vi "Connection.Properties.vi"(7 "Action":enum8{"Get", "Set"}(ring), 8 "error in (no error)":errorcluster, 10 "Connection.Properties":T1={"Server IP Address"="localhost", "Server Port"=49350, "Message Mode"=enum."None", "Security"=enum."Basic256", "User Name"="", "Password"="", "Client Certificate"=path "", "Server Certificate"=path ""}, 11 "Item Ref in":T2 format="%.0x") -> (0 "error out":errorcluster, 2 "Connection.Properties":T1={"Server IP Address"="localhost", "Server Port"=49350, "Message Mode"=enum."None", "Security"=enum."Basic256", "User Name"="", "Password"="", "Client Certificate"=path "", "Server Certificate"=path ""}, 3 "Item Ref out":T2 format="%.0x")   [LabVIEW 2013, in "OPC UA Client System Explorer.lvlib"]
uses:
  OPC UA Client System Explorer.lvlib
  <vilib>/NI Veristand/Custom Device API/Custom Device Item Ref.ctl
  Shared/Connection.Properties.ctl
  <vilib>/NI Veristand/Custom Device API/Dependent File Optional Info.ctl
  Shared/Constants.vi
  <vilib>/NI Veristand/Custom Device API/Get Item Property (String).vi
  <vilib>/NI Veristand/Custom Device API/Get Item Property (U16).vi
  <vilib>/NI Veristand/Custom Device API/Get Item Property (Dependent File).vi
  <vilib>/NI Veristand/Custom Device API/Set Item Property (String).vi
  <vilib>/NI Veristand/Custom Device API/Set Item Property (U16).vi
  <vilib>/NI Veristand/Custom Device API/Set Item Property (Dependent File).vi
  <vilib>/NI Veristand/Custom Device API/Custom Device API.lvlib
  Shared/OPC UA Client Shared.lvlib
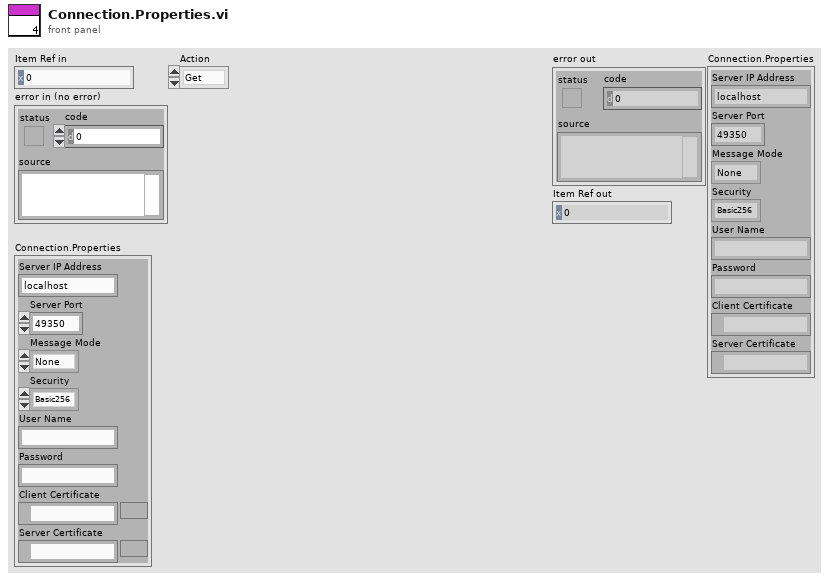
[diagram p1: front panel]
types:
  T1 = typedef "OPC UA Client Shared.lvlib/Connection.Properties.ctl" = cluster{"Server IP Address":string, "Server Port":u16, "Message Mode":enum16{"None", "Sign", "Sign and Encrypt"}, "Security":enum16{"Basic256", "Basic128Rsa15"}, "User Name":string, "Password":string, "Client Certificate":path, "Server Certificate":path}
  T2 = typedef "Custom Device API.lvlib/Custom Device Item Ref.ctl" = u64
  T3 = typedef "Custom Device API.lvlib/Dependent File Optional Info.ctl" = cluster{"Version":string, "RTDestination":path, "ForceDownload":bool, "SupportedTarget":string, "MD5":string}
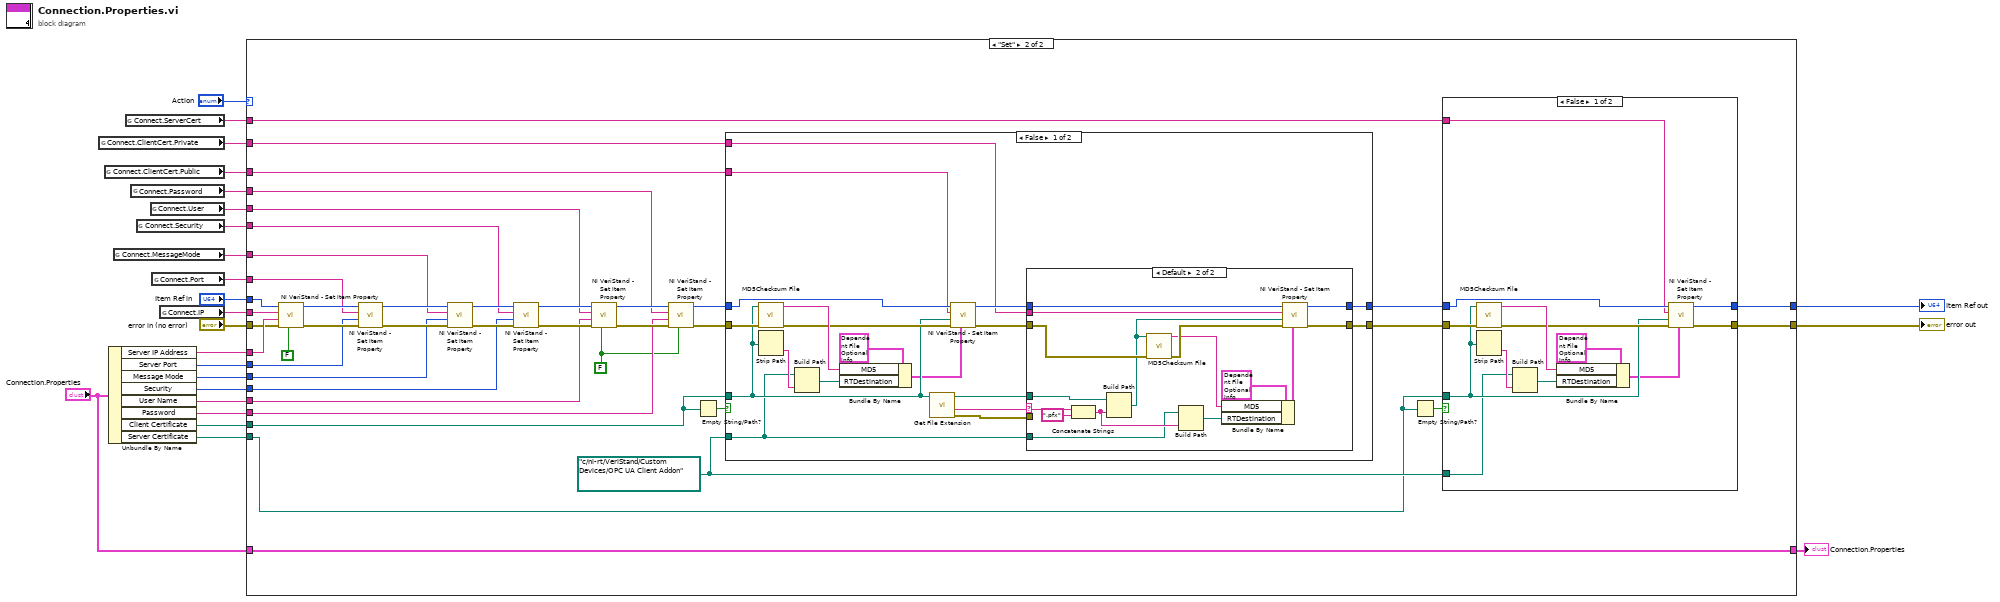
[diagram p0: block diagram]
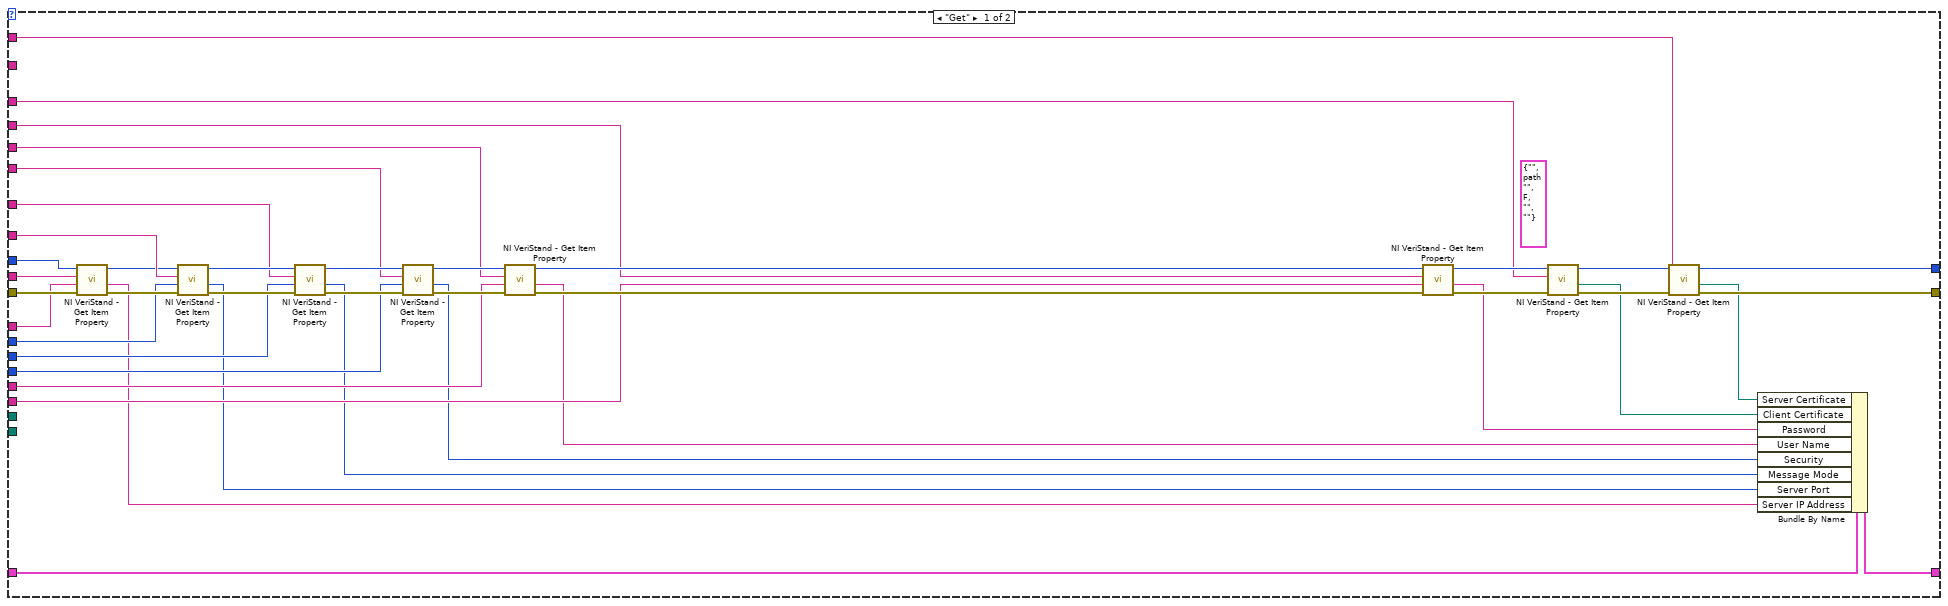
[diagram p2: hidden frame]
diagram:
  n1 = global read "Constants.vi" "Connect.ClientCert.Private"() -> (w15:string)
  n2 = global read "Constants.vi" "Connect.ClientCert.Public"() -> (w14:string)
  n3 = Unbundle By Name("Connection.Properties") -> ("Server IP Address"=w23:string, "Server Port"=w22:u16, "Message Mode"=w21:enum16{"None", "Sign", "Sign and Encrypt"}, "Security"=w20:enum16{"Basic256", "Basic128Rsa15"}, "User Name"=w19:string, "Password"=w18:string, "Client Certificate"=w4:path, "Server Certificate"=w17:path)
  n4 = global read "Constants.vi" "Connect.MessageMode"() -> (w12:string)
  n5 = global read "Constants.vi" "Connect.ServerCert"() -> (w16:string)
  n6 = global read "Constants.vi" "Connect.Password"() -> (w10:string)
  n7 = global read "Constants.vi" "Connect.Security"() -> (w13:string)
  n8 = global read "Constants.vi" "Connect.User"() -> (w11:string)
  n9 = global read "Constants.vi" "Connect.Port"() -> (w5:string)
  n10 = global read "Constants.vi" "Connect.IP"() -> (w24:string)
  n11 = case shown="\"Set\"" "Action" {
    tunnel: w24 -> [w57 w107]
    tunnel: w23 -> [w48 w94]
    tunnel: w22 -> [w47 w93]
    tunnel: w21 -> [w46 w92]
    tunnel: w20 -> [w45 w91]
    tunnel: w19 -> [w44 w90]
    tunnel: w18 -> [w43 w89]
    tunnel: w17 -> [_ w67]
    tunnel: w16 -> [w35 w72]
    tunnel: w15 -> [_ w88]
    tunnel: w14 -> [w36 w87]
    tunnel: w13 -> [w39 w86]
    tunnel: w12 -> [w40 w85]
    tunnel: w11 -> [w38 w84]
    tunnel: w10 -> [w37 w83]
    tunnel: [w42 w70] -> w9
    tunnel: [w41 w71] -> w8
    tunnel: "Item Ref in" -> [w58 w80]
    tunnel: "error in (no error)" -> [w66 w79]
    tunnel: w5 -> [w56 w78]
    tunnel: w4 -> [_ w76]
    tunnel: "Connection.Properties" -> [w34 w77]
    tunnel: [w25 w77] -> w2
    frame "Get" {
      (unwired) T3 {"Version"="", "RTDestination"=path "", "ForceDownload"=FALSE, "SupportedTarget"="", "MD5"=""} ("OptionalInfo")
      n12 = call-poly <vilib>:"NI VeriStand - Get Item Property.vi"("error in (no error)"=w66, "Default Value"=w48, "Property Name"=w57, "Item Ref in"=w58) -> ("error out"=w65:errorcluster, "Value"=w29:string, "Item Ref out"=w55:T2)  [unwired: 4 in, 1 out]
      n13 = call-poly <vilib>:"NI VeriStand - Get Item Property.vi"("error in (no error)"=w65, "Default Value"=w47, "Property Name"=w56, "Item Ref in"=w55) -> ("error out"=w64:errorcluster, "Value"=w28:u16, "Item Ref out"=w54:T2)  [unwired: 4 in, 1 out]
      n14 = call-poly <vilib>:"NI VeriStand - Get Item Property.vi"("error in (no error)"=w64, "Default Value"=w46, "Property Name"=w40, "Item Ref in"=w54) -> ("error out"=w63:errorcluster, "Value"=w27:u16, "Item Ref out"=w53:T2)  [unwired: 4 in, 1 out]
      n15 = call-poly <vilib>:"NI VeriStand - Get Item Property.vi"("error in (no error)"=w63, "Default Value"=w45, "Property Name"=w39, "Item Ref in"=w53) -> ("error out"=w62:errorcluster, "Value"=w26:u16, "Item Ref out"=w52:T2)  [unwired: 4 in, 1 out]
      n16 = call-poly <vilib>:"NI VeriStand - Get Item Property.vi"("error in (no error)"=w62, "Default Value"=w44, "Property Name"=w38, "Item Ref in"=w52) -> ("error out"=w61:errorcluster, "Value"=w30:string, "Item Ref out"=w51:T2)  [unwired: 4 in, 1 out]
      n17 = call-poly <vilib>:"NI VeriStand - Get Item Property.vi"("error in (no error)"=w61, "Default Value"=w43, "Property Name"=w37, "Item Ref in"=w51) -> ("error out"=w60:errorcluster, "Value"=w31:string, "Item Ref out"=w50:T2)  [unwired: 4 in, 1 out]
      n18 = call-poly <vilib>:"NI VeriStand - Get Item Property.vi"("error in (no error)"=w60, "Property Name"=w36, "Item Ref in"=w50) -> ("error out"=w59:errorcluster, "Path"=w32:path, "Item Ref out"=w49:T2)  [unwired: 4 in, 2 out]
      n19 = call-poly <vilib>:"NI VeriStand - Get Item Property.vi"("error in (no error)"=w59, "Property Name"=w35, "Item Ref in"=w49) -> ("error out"=w42:errorcluster, "Path"=w33:path, "Item Ref out"=w41:T2)  [unwired: 4 in, 2 out]
      n20 = Bundle By Name(cluster=w34, "Server Certificate"=w33, "Client Certificate"=w32, "Password"=w31, "User Name"=w30, "Security"=w26, "Message Mode"=w27, "Server Port"=w28, "Server IP Address"=w29) -> (w25:T1)
    }
    frame "Set" {
      w69 = path "c:/ni-rt/VeriStand/Custom Devices/OPC UA Client Addon" ("RTDestination")
      w82 = FALSE ("Binary String (T)")
      n21 = call-poly <vilib>:"NI VeriStand - Set Item Property.vi"("Binary String (T)"=FALSE, "error in (no error)"=w79, "Value"=w94, "Property Name"=w107, "Item Ref in"=w80) -> ("error out"=w100:errorcluster, "Item Ref out"=w106:T2)  [unwired: 4 in, 1 out]
      n22 = call-poly <vilib>:"NI VeriStand - Set Item Property.vi"("error in (no error)"=w100, "Value"=w93, "Property Name"=w78, "Item Ref in"=w106) -> ("error out"=w99:errorcluster, "Item Ref out"=w105:T2)  [unwired: 5 in, 1 out]
      n23 = call-poly <vilib>:"NI VeriStand - Set Item Property.vi"("error in (no error)"=w99, "Value"=w92, "Property Name"=w85, "Item Ref in"=w105) -> ("error out"=w98:errorcluster, "Item Ref out"=w104:T2)  [unwired: 5 in, 1 out]
      n24 = call-poly <vilib>:"NI VeriStand - Set Item Property.vi"("error in (no error)"=w98, "Value"=w91, "Property Name"=w86, "Item Ref in"=w104) -> ("error out"=w97:errorcluster, "Item Ref out"=w103:T2)  [unwired: 5 in, 1 out]
      n25 = call-poly <vilib>:"NI VeriStand - Set Item Property.vi"("Binary String (T)"=w82, "error in (no error)"=w97, "Value"=w90, "Property Name"=w84, "Item Ref in"=w103) -> ("error out"=w96:errorcluster, "Item Ref out"=w102:T2)  [unwired: 4 in, 1 out]
      n26 = call-poly <vilib>:"NI VeriStand - Set Item Property.vi"("Binary String (T)"=w82, "error in (no error)"=w96, "Value"=w89, "Property Name"=w83, "Item Ref in"=w102) -> ("error out"=w95:errorcluster, "Item Ref out"=w101:T2)  [unwired: 4 in, 1 out]
      n27 = Empty String/Path?(string/path=w76) -> (empty?=w75:bool)
      n28 = case shown="False" w75 {
        tunnel: w101 -> [w141 w160]
        tunnel: w95 -> [w127 w161]
        tunnel: [w139 w160] -> w73
        tunnel: w88 -> [w138 _]
        tunnel: w87 -> [w137 _]
        tunnel: [w135 w161] -> w74
        tunnel: w76 -> [w125 _]
        tunnel: w69 -> [w123 _]
        frame False {
          n29 = call <vilib>:"MD5Checksum File.vi"("error in (no error)"=w127, "Path"=w125) -> ("error out"=w126:errorcluster, "MD5 message-digest"=w128:string)  [unwired: 8 in]
          n30 = Strip Path(path=w125) -> (name=w130:string)  [unwired: 1 out]
          n31 = Build Path(base path=w123, name or relative path=w130) -> (appended path=w131:path)
          n32 = Bundle By Name(cluster=T3 {"Version"="1.0", "RTDestination"=path "c:/ni-rt/VeriStand/Custom Devices/FPGA Addon", "ForceDownload"=FALSE, "SupportedTarget"="All", "MD5"=""} ("OptionalInfo"), "MD5"=w128, "RTDestination"=w131) -> (w124:T3)
          n33 = call <vilib>:"Get File Extension.vi"("file"=w125) -> ("error out"=w133:errorcluster, "filename without extension"=w134:string, "dup file"=w132:path)  [unwired: 7 in, 1 out]
          n34 = call-poly <vilib>:"NI VeriStand - Set Item Property.vi"("OptionalInfo"=w124, "error in (no error)"=w126, "Path"=w125, "Property Name"=w137, "Item Ref in"=w141) -> ("error out"=w136:errorcluster, "Item Ref out"=w140:T2)  [unwired: 4 in, 1 out]
          n35 = case shown="Default" w134 {
            selector: w134 -> [_ w155]
            tunnel: w140 -> [w142 w159]
            tunnel: [w142 w158] -> w139
            tunnel: w138 -> [_ w157]
            tunnel: w136 -> [w143 w152]
            tunnel: [w143 w156] -> w135
            tunnel: w133 -> [_ _]
            tunnel: w132 -> [_ w153]
            tunnel: w123 -> [_ w144]
            frame "" {
            }
            frame Default {
              n36 = Concatenate Strings(w155, ".pfx" ("string")) -> (w145:string)
              n37 = Build Path(base path=w153, name or relative path=w145) -> (appended path=w146:path)
              n38 = call <vilib>:"MD5Checksum File.vi"("error in (no error)"=w152, "Path"=w146) -> ("error out"=w151:errorcluster, "MD5 message-digest"=w148:string)  [unwired: 8 in]
              n39 = Build Path(base path=w144, name or relative path=w145) -> (appended path=w149:path)
              n40 = Bundle By Name(cluster=T3 {"Version"="1.0", "RTDestination"=path "c:/ni-rt/VeriStand/Custom Devices/FPGA Addon", "ForceDownload"=FALSE, "SupportedTarget"="All", "MD5"=""} ("OptionalInfo"), "MD5"=w148, "RTDestination"=w149) -> (w147:T3)
              n41 = call-poly <vilib>:"NI VeriStand - Set Item Property.vi"("OptionalInfo"=w147, "error in (no error)"=w151, "Path"=w146, "Property Name"=w157, "Item Ref in"=w159) -> ("error out"=w156:errorcluster, "Item Ref out"=w158:T2)  [unwired: 4 in, 1 out]
            }
          }
        }
        frame True {
        }
      }
      n42 = Empty String/Path?(string/path=w67) -> (empty?=w68:bool)
      n43 = case shown="False" w68 {
        tunnel: w73 -> [w120 w121]
        tunnel: w74 -> [w114 w122]
        tunnel: w72 -> [w119 _]
        tunnel: w67 -> [w112 _]
        tunnel: w69 -> [w110 _]
        tunnel: [w109 w121] -> w71
        tunnel: [w108 w122] -> w70
        frame False {
          n44 = call <vilib>:"MD5Checksum File.vi"("error in (no error)"=w114, "Path"=w112) -> ("error out"=w113:errorcluster, "MD5 message-digest"=w115:string)  [unwired: 8 in]
          n45 = Strip Path(path=w112) -> (name=w117:string)  [unwired: 1 out]
          n46 = Build Path(base path=w110, name or relative path=w117) -> (appended path=w118:path)
          n47 = Bundle By Name(cluster=T3 {"Version"="1.0", "RTDestination"=path "c:/ni-rt/VeriStand/Custom Devices/FPGA Addon", "ForceDownload"=FALSE, "SupportedTarget"="All", "MD5"=""} ("OptionalInfo"), "MD5"=w115, "RTDestination"=w118) -> (w111:T3)
          n48 = call-poly <vilib>:"NI VeriStand - Set Item Property.vi"("OptionalInfo"=w111, "error in (no error)"=w113, "Path"=w112, "Property Name"=w119, "Item Ref in"=w120) -> ("error out"=w108:errorcluster, "Item Ref out"=w109:T2)  [unwired: 4 in, 1 out]
        }
        frame True {
        }
      }
    }
  }
  "error out" <- w9
  "Item Ref out" <- w8
  "Connection.Properties" <- w2
